vi "Read Global Debug Level.vi"(8 "error in (no error)":errorcluster, 11 "Registry in":refnum<class "Registry.lvclass">) -> (0 "error out":errorcluster, 2 "Debug Level":T1, 3 "Registry out":refnum<class "Registry.lvclass">)   [LabVIEW 2025, in "LV Logging.lvlib" / "Registry.lvclass"]
uses:
  Registry.lvclass
  Type Defs/Debug Level.ctl
  Registry.lvclass/Registry.ctl
  LV Logging.lvlib
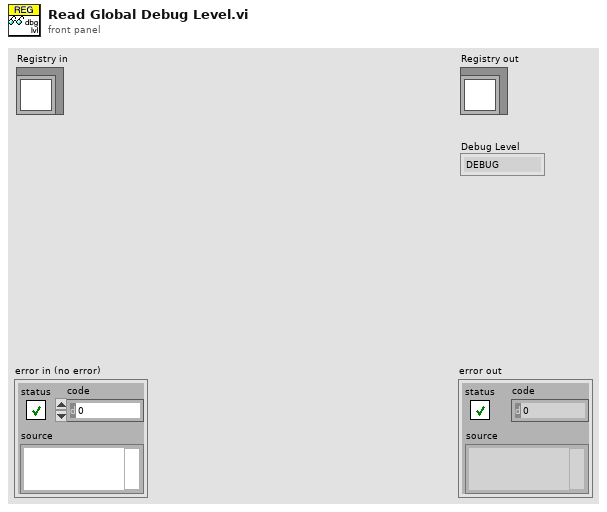
[diagram p1: front panel]
types:
  T1 = typedef "LV Logging.lvlib/Debug Level.ctl" = enum16{"DEBUG", "INFO", "WARN", "ERROR", "FATAL"}
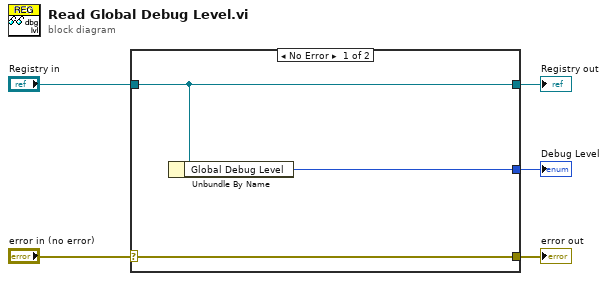
[diagram p0: block diagram]
diagram:
  n1 = case shown="No Error" "error in (no error)" {
    selector: "error in (no error)" -> [w8 w9]
    tunnel: [w8 w9] -> w4
    tunnel: [w7 w10] -> w2
    tunnel: "Registry in" -> [w7 w10]
    tunnel: [w6 _] -> w1
    frame No Error {
      n2 = Unbundle By Name(w7) -> ("Global Debug Level"=w6:T1)
    }
    frame Error {
    }
  }
  "error out" <- w4
  "Registry out" <- w2
  "Debug Level" <- w1
